vi "Obtain Request Events.vi"(8 "error in":errorcluster, 10 "Create New? (F)":bool) -> (0 "error out":errorcluster, 2 "Test Unit Request Events":T1)   [LabVIEW 2019, in "Test Unit.lvlib"]
doc: "This VI Obtains/Creates the Requests events that will be used for other modules to communicate with the module that owns this VI. These Requests events will be accessed only via Public API methods for this module.\n\n<b>NOTE</b>: The contents of this VI are automatically generated and modified by the <b>Tools > DQMH Consortium > DQMH</b> utilities. Consider using those utilities instead of making your own modifications to this VI.\n_____\nBased on DQMH Project Template 7.0.1.1316."
uses:
  Test Unit.lvlib
  Request Events--cluster.ctl
  Stop Argument--cluster.ctl
  Show Panel Argument--cluster.ctl
  Hide Panel Argument--cluster.ctl
  Show Diagram Argument--cluster.ctl
  Get Module Execution Status Argument--cluster.ctl
  TileWindows Argument--cluster.ctl
  TitleWindows Argument--cluster.ctl
  Cofiguration Argument--cluster.ctl
  <vilib>/Test Bench Framework/Test Executive.lvlibp/TestEngine/TestEngine/TestEngine/Typedefs/TestEngine Cofiguration.ctl
  <vilib>/Test Bench Framework/Test Executive.lvlibp/TestEngine/TestEngine/TestEngine/Typedefs/Local Report Configuration.ctl
  <vilib>/Test Bench Framework/Test Executive.lvlibp/TestEngine/TestEngine/TestEngine/Report Format.ctl
  <vilib>/Test Bench Framework/Test Executive.lvlibp/TestEngine/TestEngine/TestEngine/Typedefs/Database Configuration.ctl
  Load Sequence Argument--cluster.ctl
  Write SN Argument--cluster.ctl
  UUT Test Argument--cluster.ctl
  UUTs Test Argument--cluster.ctl
  Terminate Test Argument--cluster.ctl
  Set Variable Argument--cluster.ctl
  Get Variable Argument--cluster.ctl
  Get Variable (Reply Payload)--cluster.ctl
  <vilib>/Test Bench Framework/Test Executive.lvlibp/TestEngine/TestEngine/TestEngine/Test Engine.lvclass
panel:
  # "NOTE: The contents of this VI are automatically generated and modified by the Tools > DQMH Consortium > DQMH utilities. Consider using those utilities instead of making your own modifications to this VI."
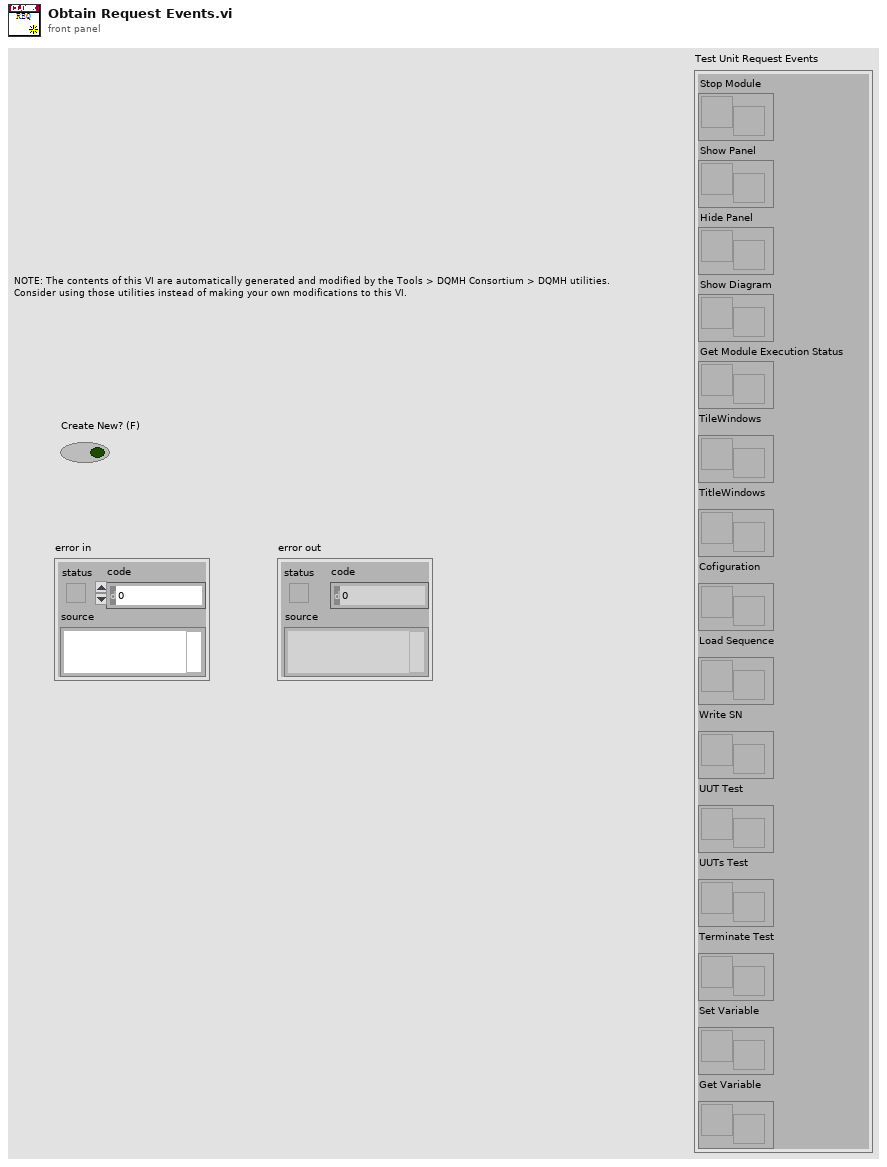
[diagram p1: front panel]
types:
  T1 = typedef "Test Unit.lvlib/Request Events--cluster.ctl" = cluster{"Stop Module":refnum<user-event>, "Show Panel":refnum<user-event>, "Hide Panel":refnum<user-event>, "Show Diagram":refnum<user-event>, "Get Module Execution Status":refnum<user-event>, "TileWindows":refnum<user-event>, "TitleWindows":refnum<user-event>, "Cofiguration":refnum<user-event>, "Load Sequence":refnum<user-event>, "Write SN":refnum<user-event>, "UUT Test":refnum<user-event>, "UUTs Test":refnum<user-event>, "Terminate Test":refnum<user-event>, "Set Variable":refnum<user-event>, "Get Variable":refnum<user-event>}
  T2 = typedef "Test Unit.lvlib/Get Variable Argument--cluster.ctl" = cluster{"Module ID":i32, "Socket":i32, "Variable":string, "Wait Notifier":refnum<notifier>, "wait for reply":bool}
  T3 = typedef "Test Unit.lvlib/Set Variable Argument--cluster.ctl" = cluster{"Module ID":i32, "Variable":string, "Socket":i32, "Value":variant}
  T4 = typedef "Test Unit.lvlib/Terminate Test Argument--cluster.ctl" = cluster{"Module ID":i32, "Abort VI":bool}
  T5 = typedef "Test Unit.lvlib/UUTs Test Argument--cluster.ctl" = cluster{"Module ID":i32, "Enable Socket":bool[]}
  T6 = typedef "Test Unit.lvlib/UUT Test Argument--cluster.ctl" = cluster{"Module ID":i32, "Socket":i32}
  T7 = typedef "Test Unit.lvlib/Write SN Argument--cluster.ctl" = cluster{"Module ID":i32, "Socket":i32, "Serial Number":string}
  T8 = typedef "Test Unit.lvlib/Load Sequence Argument--cluster.ctl" = cluster{"Module ID":i32, "File Pathname":path, "Sequence":string}
  T9 = typedef "Test Unit.lvlib/Cofiguration Argument--cluster.ctl" = cluster{"Module ID":i32, "TestEngine Cofiguration":T10}
  T10 = typedef "Test Executive.lvlibp/Test Engine.lvlib/Test Engine.lvclass/TestEngine Cofiguration.ctl" = cluster{"Break on Failure":bool, "Automatically handle TestVI error":cluster{"Enable":bool, "Handle":enum16{"Termination test", "Ignore error"}}, "Local Report Configuration":T11, "Database Configuration":T13, "Ignore breakpoint":bool, "Filter Result":bool}
  T11 = typedef "Test Executive.lvlibp/Test Engine.lvlib/Test Engine.lvclass/Local Report Configuration.ctl" = cluster{"Report Folder Path":path, "Format":T12, "Disable":bool, "Build Date Folder?":bool, "Execl Template Path":path}
  T12 = typedef "Test Executive.lvlibp/Test Engine.lvlib/Test Engine.lvclass/Report Format.ctl" = enum16{"Excel", "CSV(Tab)", "CSV(,)", "CSV(;)", "TEXT", "HTML"}
  T13 = typedef "Test Executive.lvlibp/Test Engine.lvlib/Test Engine.lvclass/Database Configuration.ctl" = cluster{"Connection String Expression":string, "Microsoft Data Link File":path, "Connection Type":enum16{"Use Connection String Expression", "Use Microsoft Data Link File"}, "Enable":bool}
  T14 = typedef "Test Unit.lvlib/TitleWindows Argument--cluster.ctl" = cluster{"Module ID":i32, "TitleWindows":bool, "dont initi":bool}
  T15 = typedef "Test Unit.lvlib/TileWindows Argument--cluster.ctl" = cluster{"Module ID":i32, "TileWindows":bool}
  T16 = typedef "Test Unit.lvlib/Get Module Execution Status Argument--cluster.ctl" = cluster{"Module ID":i32, "Running?":bool}
  T17 = typedef "Test Unit.lvlib/Show Diagram Argument--cluster.ctl" = cluster{"Module ID":i32, "Debug?":bool}
  T18 = typedef "Test Unit.lvlib/Show Panel Argument--cluster.ctl" = cluster{"Module ID":i32, "Show Panel?":bool}
  T19 = typedef "Test Unit.lvlib/Hide Panel Argument--cluster.ctl" = cluster{"Module ID":i32, "Hide Panel?":bool}
  T20 = typedef "Test Unit.lvlib/Stop Argument--cluster.ctl" = cluster{"Module ID":i32, "Origin":string, "Exit via Stop Module Req?":bool, "Wait for Module to stop?":bool}
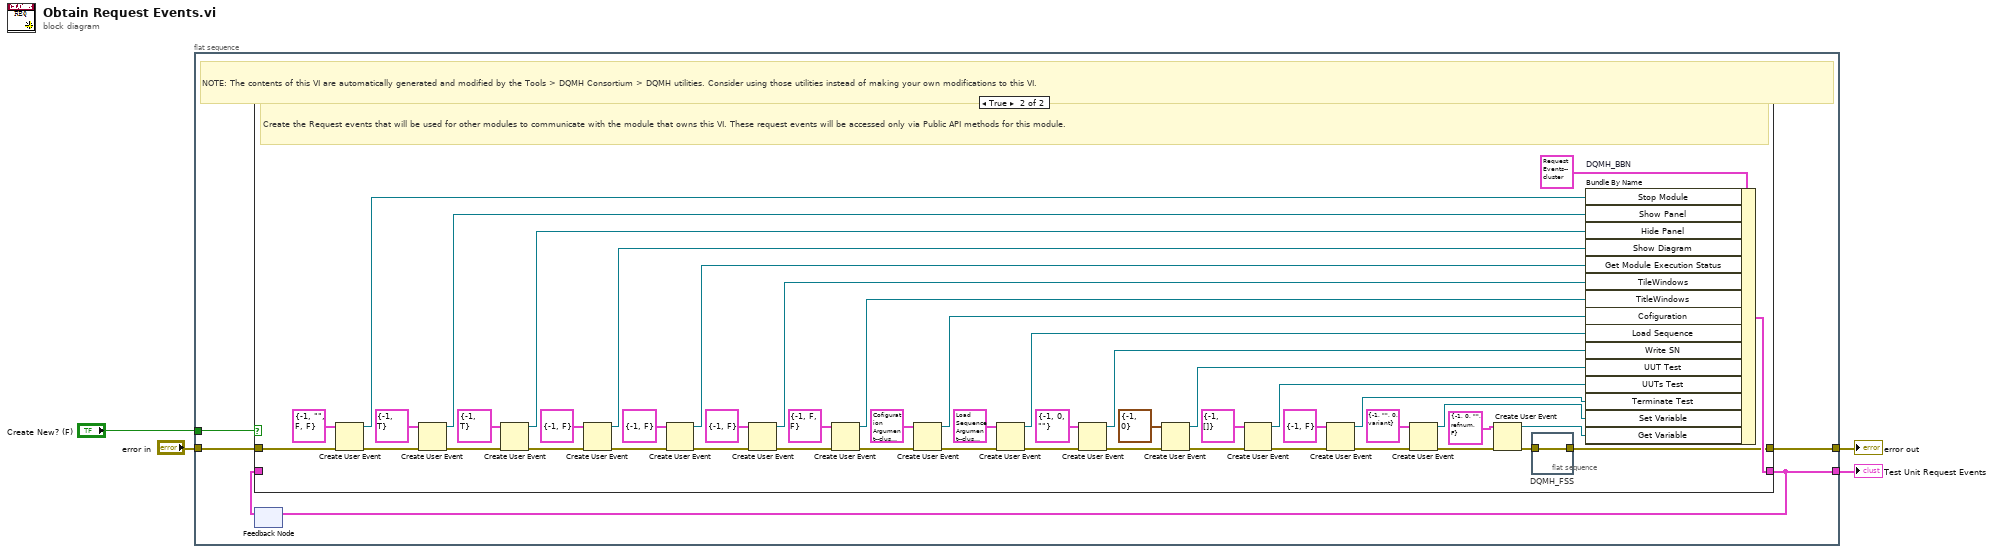
[diagram p0: block diagram]
diagram:
  n1 = flat-sequence {
    tunnel: [w9] -> w4
    tunnel: "error in" -> [w8]
    tunnel: [w6] -> w2
    tunnel: "Create New? (F)" -> [w5]
    frame #0 {
      # "NOTE: The contents of this VI are automatically generated and modified by the Tools > DQMH Consortium > DQMH utilities. Consider using those utilities instead of making your own modifications to this VI."
      n2 = feedback #1() -> (w7:T1)  [unwired: 1 in]
      n3 = case shown="True" w5 {
        tunnel: [w10 w48] -> w9
        tunnel: w8 -> [w10 w60]
        tunnel: [w11 w57] -> w6
        tunnel: w7 -> [w11 _]
        frame False {
        }
        frame True {
          # "Create the Request events that will be used for other modules to communicate with the module that owns this VI. These request events will be accessed only via Public API methods for this module."
          n4 = Create User Event(user event datatype=T20 {"Module ID"=-1, "Origin"="", "Exit via Stop Module Req?"=FALSE, "Wait for Module to stop?"=FALSE} ("Stop Argument"), error in=w60) -> (user event=w58:refnum<user-event>, error out=w55:errorcluster)
          n5 = Create User Event(user event datatype=T18 {"Module ID"=-1, "Show Panel?"=TRUE} ("Show Panel Argument"), error in=w55) -> (user event=w54:refnum<user-event>, error out=w52:errorcluster)
          n6 = Create User Event(user event datatype=T19 {"Module ID"=-1, "Hide Panel?"=TRUE} ("Hide Panel"), error in=w52) -> (user event=w51:refnum<user-event>, error out=w50:errorcluster)
          n7 = Create User Event(user event datatype=T17 {"Module ID"=-1, "Debug?"=FALSE} ("Show Diagram Argument"), error in=w50) -> (user event=w46:refnum<user-event>, error out=w47:errorcluster)
          n8 = Create User Event(user event datatype=T16 {"Module ID"=-1, "Running?"=FALSE} ("Get Module Execution Status Argument"), error in=w47) -> (user event=w43:refnum<user-event>, error out=w44:errorcluster)
          n9 = Create User Event(user event datatype=T15 {"Module ID"=-1, "TileWindows"=FALSE} ("TileWindows Argument"), error in=w44) -> (user event=w40:refnum<user-event>, error out=w41:errorcluster)
          n10 = Create User Event(user event datatype=T14 {"Module ID"=-1, "TitleWindows"=FALSE, "dont initi"=FALSE} ("TitleWindows Argument"), error in=w41) -> (user event=w37:refnum<user-event>, error out=w38:errorcluster)
          n11 = Create User Event(user event datatype=T9 {"Module ID"=-1, "TestEngine Cofiguration"={"Break on Failure"=FALSE, "Automatically handle TestVI error"={"Enable"=FALSE, "Handle"=enum."Termination test"}, "Local Report Configuration"={"Report Folder Path"=path "", "Format"=enum."Excel", "Disable"=FALSE, "Build Date Folder?"=FALSE, "Execl Template Path"=path ""}, "Database Configuration"={"Connection String Expression"="", "Microsoft Data Link File"=path "", "Connection Type"=enum."Use Connection String Expression", "Enable"=FALSE}, "Ignore breakpoint"=FALSE, "Filter Result"=FALSE}} ("Cofiguration Argument"), error in=w38) -> (user event=w34:refnum<user-event>, error out=w35:errorcluster)
          n12 = Create User Event(user event datatype=T8 {"Module ID"=-1, "File Pathname"=path "", "Sequence"="Main_Sequence"} ("Load Sequence Argument"), error in=w35) -> (user event=w31:refnum<user-event>, error out=w32:errorcluster)
          n13 = Create User Event(user event datatype=T7 {"Module ID"=-1, "Socket"=0, "Serial Number"=""} ("Write SN Argument"), error in=w32) -> (user event=w28:refnum<user-event>, error out=w29:errorcluster)
          n14 = Create User Event(user event datatype=T6 {"Module ID"=-1, "Socket"=0} ("UUT Test Argument"), error in=w29) -> (user event=w25:refnum<user-event>, error out=w26:errorcluster)
          n15 = Create User Event(user event datatype=T5 {"Module ID"=-1, "Enable Socket"=[]} ("UUTs Test Argument"), error in=w26) -> (user event=w22:refnum<user-event>, error out=w23:errorcluster)
          n16 = Create User Event(user event datatype=T4 {"Module ID"=-1, "Abort VI"=FALSE} ("Terminate Test Argument"), error in=w23) -> (user event=w19:refnum<user-event>, error out=w20:errorcluster)
          n17 = Create User Event(user event datatype=T3 {"Module ID"=-1, "Variable"="", "Socket"=0, "Value"=variant} ("Set Variable Argument"), error in=w20) -> (user event=w16:refnum<user-event>, error out=w17:errorcluster)
          n18 = Create User Event(user event datatype=T2 {"Module ID"=-1, "Socket"=0, "Variable"="", "Wait Notifier"=refnum, "wait for reply"=FALSE} ("Get Variable Argument"), error in=w17) -> (user event=w13:refnum<user-event>, error out=w14:errorcluster)
          n19 = flat-sequence "DQMH_FSS" {
            tunnel: w14 -> [w61]
            tunnel: [w61] -> w48
            frame #0 {
            }
          }
          n20 = Bundle By Name "DQMH_BBN"(cluster=T1 {"Stop Module"=refnum, "Show Panel"=refnum, "Hide Panel"=refnum, "Show Diagram"=refnum, "Get Module Execution Status"=refnum, "TileWindows"=refnum, "TitleWindows"=refnum, "Cofiguration"=refnum, "Load Sequence"=refnum, "Write SN"=refnum, "UUT Test"=refnum, "UUTs Test"=refnum, "Terminate Test"=refnum, "Set Variable"=refnum, "Get Variable"=refnum} ("output cluster"), "Stop Module"=w58, "Show Panel"=w54, "Hide Panel"=w51, "Show Diagram"=w46, "Get Module Execution Status"=w43, "TileWindows"=w40, "TitleWindows"=w37, "Cofiguration"=w34, "Load Sequence"=w31, "Write SN"=w28, "UUT Test"=w25, "UUTs Test"=w22, "Terminate Test"=w19, "Set Variable"=w16, "Get Variable"=w13) -> (w57:T1)
        }
      }
      n21 = feedback-in #1(w6) -> ()
    }
  }
  "Test Unit Request Events" <- w2
  "error out" <- w4
